vi "Main.vi"(11 "Module Admin":refnum<class "Delacor_lib_QMH_Module Admin.lvclass">) -> ()   [LabVIEW 2020, in "UI.lvlib"]
doc: "This template is based off of the Queued Message Handler design pattern and the Queued Message Handler project template that ships with LabVIEW.\n\nThe main difference is that the queue is private to this module and communication between modules is performed via Broadcast and Request events.\n\nRequest events are wrapped in public API methods and are handled in the Event Handling Loop (EHL) of this VI. Any module can register for Broadcast events sent by this module. The EHL generates messages based on user interface actions.\n\nThe Message Handling Loop (MHL) processes messages generated by the EHL, or by other messages. The messages are string values, so new messages can be added easily to the Message Cases case structure in the MHL. Each message cluster can also provide an optional value for Message Data, which is a variant that can be converted to whatever message-specific data is required.\n_____\nBased on Delacor QMH Project Template 5.0.0.82."
uses:
  UI.lvlib
  <vilib>/Delacor/Delacor QMH/Libraries/Module Admin_class/Delacor_lib_QMH_Module Admin.lvclass
  Module Data--cluster.ctl
  Stop Argument--cluster.ctl
  <vilib>/Delacor/Delacor QMH/Libraries/Message Queue_class/Delacor_lib_QMH_Message Queue.lvclass/Delacor_lib_QMH_Message Queue.ctl
  <vilib>/Delacor/Delacor QMH/Libraries/Module Admin_class/Delacor_lib_QMH_Module Admin.lvclass/Delacor_lib_QMH_Module Admin.ctl
  <vilib>/Utility/miscctls.llb/LVPointTypeDef.ctl
  <vilib>/Delacor/Delacor QMH/Libraries/Message Queue_class/Delacor_lib_QMH_Enqueue Message (Single).vi
  <vilib>/Delacor/Delacor QMH/Libraries/Module Admin_class/Delacor_lib_QMH_Get External Launch.vi
  <vilib>/Utility/error.llb/Error Cluster From Error Code.vi
  <vilib>/ErrorRing/Error Ring.xnode
  <vilib>/Delacor/Delacor QMH/Libraries/Message Queue_class/Delacor_lib_QMH_Message Queue.lvclass
  Acquisition whit helper loop/Acquisition whit helper loop.lvlib
panel:
  in  "Stop Acq":bool
  in  "Start Acq":bool
  out "error out":errorcluster
  out "Status":string
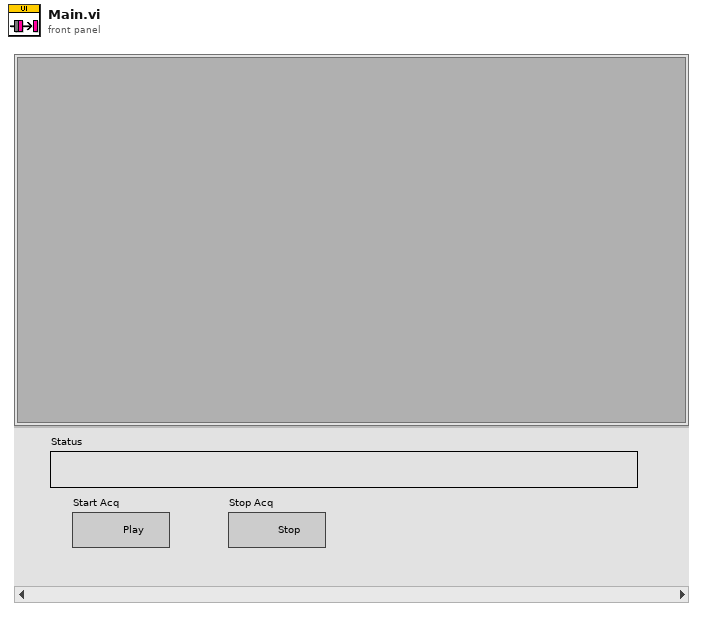
[diagram p1: front panel]
types:
  T1 = typedef "UI.lvlib/Request Events--cluster.ctl" = cluster{"Stop Module":refnum<user-event>, "Show Panel":refnum<user-event>, "Hide Panel":refnum<user-event>, "Get Module Execution Status":refnum<user-event>, "Show Diagram":refnum<user-event>}
  T2 = typedef "Acquisition whit helper loop.lvlib/Broadcast Events--cluster.ctl" = cluster{"Module Did Init":refnum<user-event>, "Status Updated":refnum<user-event>, "Error Reported":refnum<user-event>, "Module Did Stop":refnum<user-event>, "Update Module Execution Status":refnum<user-event>}
  T3 = typedef "UI.lvlib/Module Data--cluster.ctl" = cluster{"Status":string}
  T4 = enum32{"invalid lock state", "Not Locked", "Locked (No Password)", "Password-protected"}
  T5 = typedef "UI.lvlib/Stop Argument--cluster.ctl" = cluster{"Origin":string, "Exit via Stop Module Req?":bool, "Wait for Module to stop?":bool}
  T6 = enum32{"Invalid", "Standard", "Closed", "Hidden", "Minimized", "Maximized"}
  T7 = typedef "LVPointTypeDef.ctl" = cluster{"Horizontal":i16, "Vertical":i16}
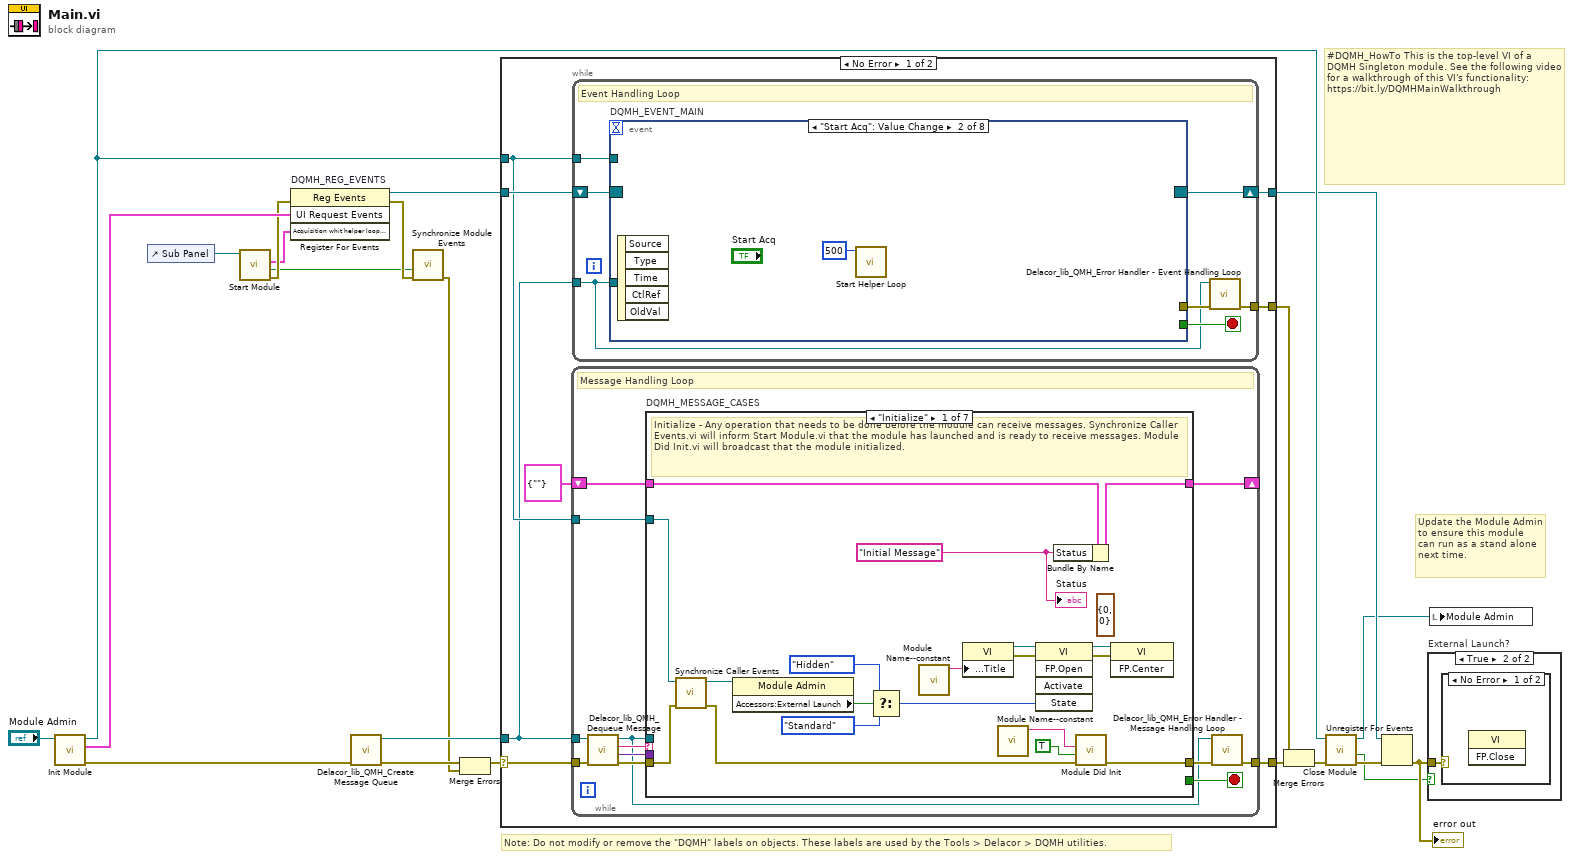
[diagram p0: block diagram]
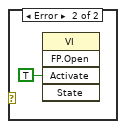
[diagram p3: hidden frame]
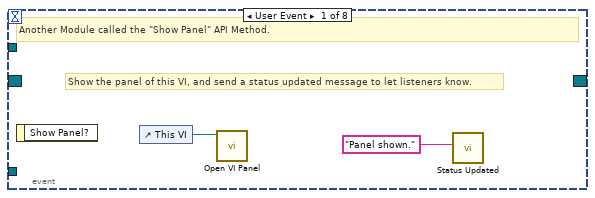
[diagram p4: hidden frame]
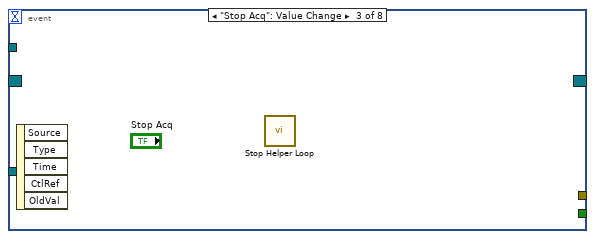
[diagram p5: hidden frame]
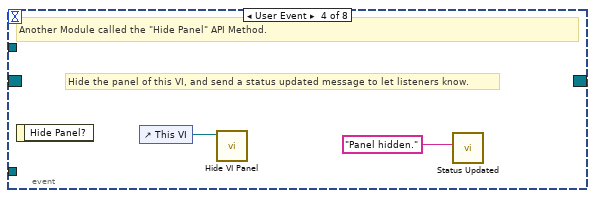
[diagram p6: hidden frame]
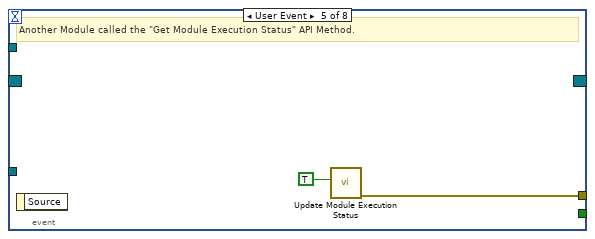
[diagram p7: hidden frame]
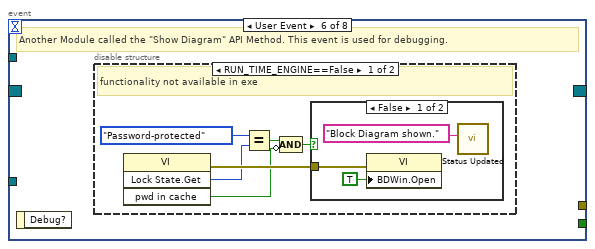
[diagram p8: hidden frame]
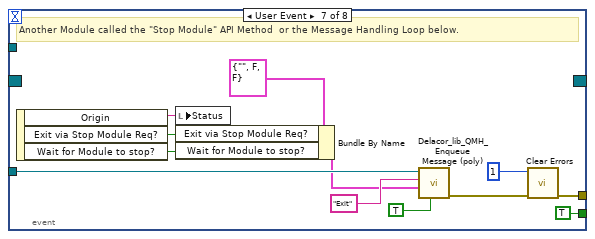
[diagram p11: hidden frame]
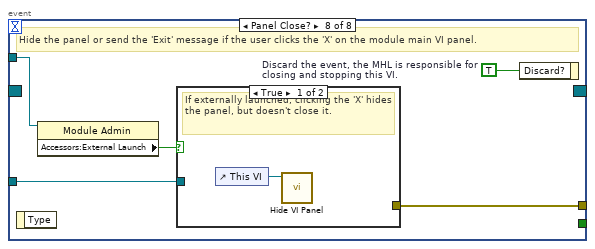
[diagram p12: hidden frame]
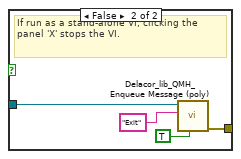
[diagram p13: hidden frame]
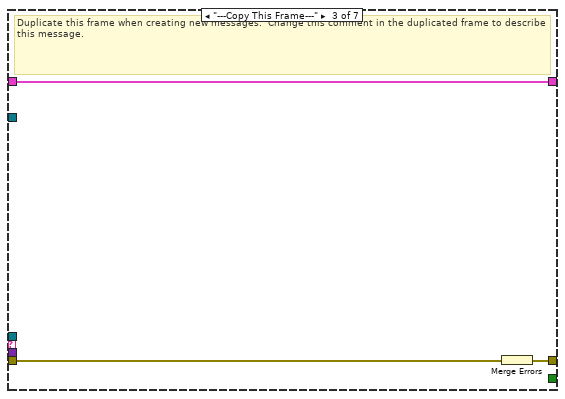
[diagram p15: hidden frame]
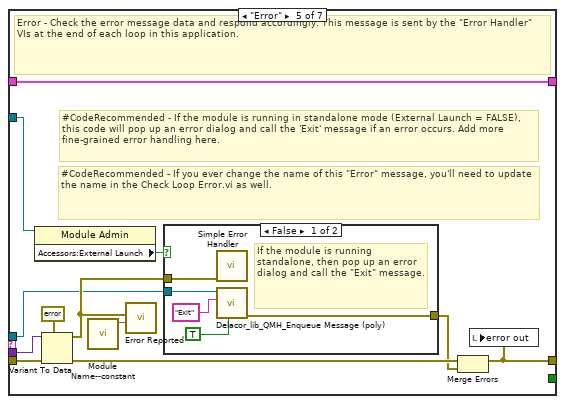
[diagram p17: hidden frame]
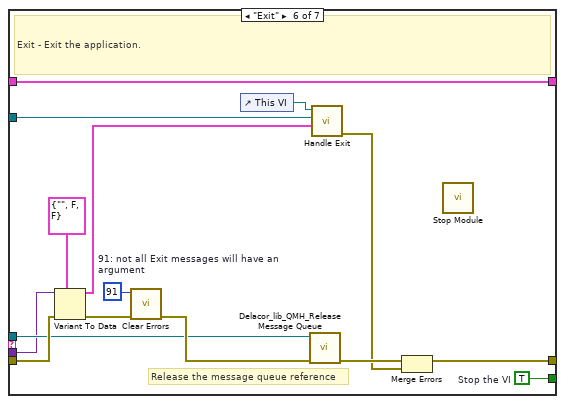
[diagram p19: hidden frame]
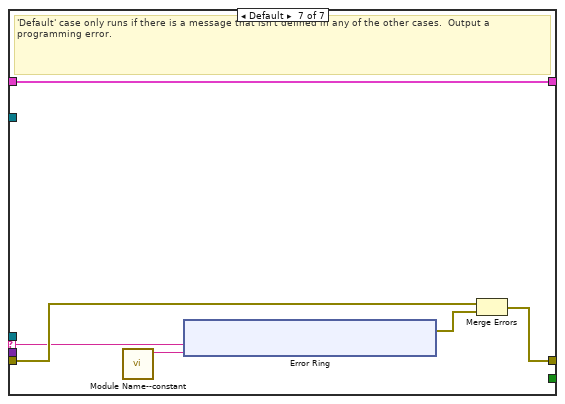
[diagram p20: hidden frame]
diagram:
  # "#DQMH_HowTo This is the top-level VI of a DQMH Singleton module. See the following video for a walkthrough of this VI's functionality: https://bit.ly/DQMHMainWalkthrough"
  # "Note: Do not modify or remove the \"DQMH\" labels on objects. These labels are used by the Tools > Delacor > DQMH utilities."
  # "Update the Module Admin to ensure this module can run as a stand alone next time."
  n1 = call "Init Module.vi"("Singleton Module Admin in"="Module Admin") -> ("error out"=w21:errorcluster, "UI Request Events"=w11:T1, "Singleton Module Admin out"=w14:refnum<class "Delacor_lib_QMH_Module Admin.lvclass">)  [unwired: 8 in]
  n2 = control-ref of="Sub Panel"() -> (w1:refnum<vi>)
  n3 = call "Start Module.vi"("Acquisition Panel"=w1) -> ("error out"=w4:errorcluster, "Wait for Event Sync?"=w3:bool, "Acquisition whit helper loop Broadcast Events"=w2:T2)  [unwired: 7 in, 1 out]
  n4 = register-events "DQMH_REG_EVENTS"(error in=w4, w11, w2) -> (reference out=w12:refnum<event-registration>, error out=w6:errorcluster)  [unwired: 1 in]
  n5 = call <vilib>:"Delacor_lib_QMH_Create Message Queue.vi"("error in (no error)"=w21) -> ("error out"=w16:errorcluster, "Message Queue"=w10:refnum<class "Delacor_lib_QMH_Message Queue.lvclass">)  [unwired: 9 in]
  n6 = call "Synchronize Module Events.vi"("error in (no error)"=w6, "Wait for Event Sync?"=w3) -> ("error out"=w5:errorcluster)  [unwired: 9 in]
  n7 = Merge Errors(w16, w5) -> (w15:errorcluster)
  n8 = case shown="No Error" w15 {
    selector: w15 -> [w28 w162]
    tunnel: [w30 w161] -> w22
    tunnel: [w27 w167] -> w13
    tunnel: w12 -> [w25 w167]
    tunnel: w10 -> [w23 w160]
    tunnel: [w29 _] -> w19
    tunnel: w14 -> [w24 w163]
    frame No Error {
      n9 = while {
        tunnel: w23 -> [w78]
        shift-right: [w82] -> _
        shift-left: T3 {"Status"=""} ("Data Cluster") -> [w83]
        tunnel: w28 -> [w86]
        tunnel: [w84] -> w30
        tunnel: w24 -> [w76]
        stop <- w81 stop-if-true
        # "Message Handling Loop"
        n10 = call-dynamic "Delacor_lib_QMH_Dequeue Message.vi"("error in (no error)"=w86, "Message Queue in"=w78) -> ("error out"=w85:errorcluster, "Message Data"=w79:variant, "Message"=w80:string, "Message Queue out"=w77:refnum<class "Delacor_lib_QMH_Message Queue.lvclass">)  [unwired: 6 in]
        n11 = case "DQMH_MESSAGE_CASES" shown="\"Initialize\"" w80 {
          selector: w80 -> [_ _ _ _ _ _ w147]
          tunnel: w77 -> [_ _ _ _ w117 w139 _]
          tunnel: w85 -> [w104 w108 w111 w113 w124 w145 w149]
          tunnel: [w102 w108 w110 w113 w120 w142 w150] -> w87
          tunnel: w83 -> [w94 w107 w109 w112 w119 w138 w148]
          tunnel: [w93 w107 w109 w112 w119 w138 w148] -> w82
          tunnel: [_ _ _ _ _ w137 _] -> w81
          tunnel: w79 -> [_ _ _ _ w118 w136 _]
          tunnel: w76 -> [w89 _ _ _ w116 w131 _]
          frame "Initialize" {
            (unwired) T7 {"Horizontal"=0, "Vertical"=0} ("Origin")
            w90 = "Initial Message" ("Initial Message")
            # "Initialize - Any operation that needs to be done before the module can receive messages. Synchronize Caller Events.vi will inform Start Module.vi that the module has launched and is ready to receive messages. Module Did Init.vi will broadcast that the module initialized."
            n12 = call "Synchronize Caller Events.vi"("error in (no error)"=w104, "Singleton Module Admin in"=w89) -> ("error out"=w103:errorcluster, "Singleton Module Admin out"=w88:refnum<class "Delacor_lib_QMH_Module Admin.lvclass">)  [unwired: 8 in]
            n13 = property class="Module Admin"(reference=w88) -> ("Accessors:External Launch"=w98:bool)  [unwired: 1 in, 2 out]
            n14 = Select(t=T6."Hidden" ("State"), s=w98, f=T6."Standard" ("State")) -> (s? t:f=w95:T6)
            n15 = call "Module Name--constant.vi"() -> ("Module Name"=w101:string)  [unwired: 11 in]
            n16 = property class="VI"("Front Panel.Title"=w101) -> (reference out=w100:refnum<vi>, error out=w106:errorcluster)  [unwired: 2 in]
            n17 = call "Module Name--constant.vi"() -> ("Module Name"=w91:string)  [unwired: 11 in]
            n18 = invoke class="VI" method="FP.Open"(reference=w100, error in=w106, "State"=w95) -> (reference out=w99:refnum<vi>, error out=w105:errorcluster)  [unwired: 2 in, 3 out]
            n19 = Bundle By Name(cluster=w94, "Status"=w90) -> (w93:T3)
            n20 = call "Module Did Init.vi"("error in (no error)"=w103, "Initialized?"=TRUE, "Origin"=w91) -> ("error out"=w102:errorcluster)  [unwired: 8 in]
            n21 = invoke class="VI" method="FP.Center"(reference=w99, error in=w105) -> ()  [unwired: 1 in, 3 out]
            "Status" <- w90
          }
          frame "--- Module Specific ---" {
            # "Separator -- The following cases handle messages specific to this Module."
          }
          frame "---Copy This Frame---" {
            # "Duplicate this frame when creating new messages.  Change this comment in the duplicated frame to describe this message."
            n22 = Merge Errors(w111) -> (w110:errorcluster)
          }
          frame "--- Exit and Error Handling---" {
            # "Separator - The following cases handle errors and exit messages."
          }
          frame "Error" {
            # "#CodeRecommended - If you ever change the name of this \"Error\" message, you'll need to update the name in the Check Loop Error.vi as well."
            # "#CodeRecommended - If the module is running in standalone mode (External Launch = FALSE), this code will pop up an error dialog and call the 'Exit' message if an error occurs. Add more fine-grained error handling here."
            # "Error - Check the error message data and respond accordingly. This message is sent by the \"Error Handler\" VIs at the end of each loop in this application."
            n23 = property class="Module Admin"(reference=w116) -> ("Accessors:External Launch"=w115:bool)  [unwired: 1 in, 2 out]
            n24 = Variant To Data(error in=w124, type=errorcluster {"status"=FALSE, "code"=0, "source"=""} ("error constant"), Variant=w118) -> (data=w125:errorcluster, error out=w122:errorcluster)
            n25 = call "Module Name--constant.vi"() -> ("Module Name"=w114:string)  [unwired: 11 in]
            n26 = call "Error Reported.vi"("Additional Information"=w114, "Error"=w125) -> ()  [unwired: 9 in, 1 out]
            n27 = case shown="False" w115 {
              tunnel: [w130 _] -> w121
              tunnel: w117 -> [w128 _]
              tunnel: w125 -> [w129 _]
              frame False {
                # "If the module is running standalone, then pop up an error dialog and call the \"Exit\" message."
                n28 = call <vilib>:"Simple Error Handler.vi"("error in (no error)"=w129) -> ()  [unwired: 4 in, 5 out]
                n29 = call-poly <vilib>:"Delacor_lib_QMH_Enqueue Message (poly).vi"("Priority Message? (F)"=TRUE, "Message"="Exit", "Message Queue in"=w128) -> ("error out"=w130:errorcluster)  [unwired: 7 in, 1 out]
              }
              frame True {
                # "If the module was launched externally, calling the Error Reported broadcast VI is the only action performed by the \"Error\" message. The module's caller can then process the error appropriately."
              }
            }
            n30 = Merge Errors(w122, w121) -> (w120:errorcluster)
            n31 = local write "error out"(w120) -> ()
          }
          frame "Exit" {
            w135 = 91  # 91: not all Exit messages will have an argument
            w137 = TRUE  # Stop the VI
            # "Release the message queue reference"
            # "Exit - Exit the application."
            n32 = Variant To Data(error in=w145, type=T5 {"Origin"="", "Exit via Stop Module Req?"=FALSE, "Wait for Module to stop?"=FALSE} ("Stop Argument"), Variant=w136) -> (data=w133:T5, error out=w141:errorcluster)
            n33 = call <vilib>:"Clear Errors.vi"("error in (no error)"=w141, "specific error code to clear (0: all)"=w135) -> ("error out"=w144:errorcluster)  [unwired: 4 in, 1 out]
            n34 = control-ref of="This VI"() -> (w132:refnum<vi>)
            n35 = call-dynamic "Delacor_lib_QMH_Release Message Queue.vi"("error in (no error)"=w144, "Message Queue"=w139) -> ("error out"=w143:errorcluster)  [unwired: 9 in]
            n36 = call "Handle Exit.vi"("Stop Argument"=w133, "Admin in"=w131, "VI reference"=w132) -> ("error out"=w140:errorcluster)  [unwired: 7 in, 1 out]
            n37 = Merge Errors(w143, w140) -> (w142:errorcluster)
            n38 = call "Stop Module.vi"() -> ()  [unwired: 11 in, 1 out]
          }
          frame Default {
            # "'Default' case only runs if there is a message that isn't defined in any of the other cases.  Output a programming error."
            n39 = call "Module Name--constant.vi"() -> ("Module Name"=w146:string)  [unwired: 11 in]
            n40 = xnode "Error Ring"("parameter 0"=w147, "parameter 1"=w146) -> ("error out"=w151:errorcluster)
            n41 = Merge Errors(w149, w151) -> (w150:errorcluster)
          }
        }
        n42 = call-dynamic "Delacor_lib_QMH_Error Handler - Message Handling Loop.vi"("error in (no error)"=w87, "Message Queue in"=w77) -> ("dup error in"=w84:errorcluster)  [unwired: 8 in, 1 out]
      }
      n43 = while {
        tunnel: w23 -> [w31]
        shift-right: [w34] -> w27
        shift-left: w25 -> [w35]
        tunnel: [w36] -> w29
        tunnel: w24 -> [w32]
        stop <- w33 stop-if-true
        # "Event Handling Loop"
        n44 = event "DQMH_EVENT_MAIN" shown="[1] \"Start Acq\": Value Change" {
          selector: w35 -> [_ _ _ _ _ _ _ _]
          dyn-events: [_ _ _ _ _ _ _ _] -> w34
          timeout: _ -> [_ _ _ _ _ _ _ _]
          tunnel: [_ _ _ _ _ _ TRUE ("Discard?") _] -> w33
          tunnel: w31 -> [_ _ _ _ _ _ w61 w68]
          tunnel: [_ _ _ _ w44 _ w64 w70] -> w37
          tunnel: w32 -> [_ _ _ _ _ _ _ w67]
          event User Event {
            # "Show the panel of this VI, and send a status updated message to let listeners know."
            # "Another Module called the \"Show Panel\" API Method."
            n45 = event-data() -> ()  [unwired: 1 in, 1 out]
            n46 = control-ref of="This VI"() -> (w39:refnum<vi>)
            n47 = call "Open VI Panel.vi"("VI"=w39) -> ()  [unwired: 10 in, 1 out]
            n48 = call "Status Updated.vi"("Status"="Panel shown." ("format string")) -> ()  [unwired: 10 in, 1 out]
          }
          event "Start Acq": Value Change {
            n49 = event-data() -> ()  [unwired: 1 in, 5 out]
            n50 = call "Start Helper Loop.vi"("Delay Timeout"=500) -> ()  [unwired: 10 in, 1 out]
          }
          event "Stop Acq": Value Change {
            n51 = event-data() -> ()  [unwired: 1 in, 5 out]
            n52 = call "Stop Helper Loop.vi"() -> ()  [unwired: 11 in, 1 out]
          }
          event User Event {
            # "Hide the panel of this VI, and send a status updated message to let listeners know."
            # "Another Module called the \"Hide Panel\" API Method."
            n53 = event-data() -> ()  [unwired: 1 in, 1 out]
            n54 = control-ref of="This VI"() -> (w42:refnum<vi>)
            n55 = call "Hide VI Panel.vi"("VI"=w42) -> ()  [unwired: 10 in, 1 out]
            n56 = call "Status Updated.vi"("Status"="Panel hidden." ("format string")) -> ()  [unwired: 10 in, 1 out]
          }
          event User Event {
            # "Another Module called the \"Get Module Execution Status\" API Method."
            n57 = event-data() -> ()  [unwired: 1 in, 1 out]
            n58 = call "Update Module Execution Status.vi"("Running?"=TRUE) -> ("error out"=w44:errorcluster)  [unwired: 10 in]
          }
          event User Event {
            # "Another Module called the \"Show Diagram\" API Method. This event is used for debugging."
            n59 = event-data() -> ()  [unwired: 1 in, 1 out]
            n60 = disable-structure shown="RUN_TIME_ENGINE==False" {
              frame condition #0 (active) {
                # "functionality not available in exe"
                n61 = invoke class="VI" method="Lock State.Get"() -> (error out=w50:errorcluster, "Get Lock State"=w49:T4, "pwd in cache"=w46:bool)  [unwired: 4 in, 1 out]
                n62 = Equal?(x=T4."Password-protected", y=w49) -> (x = y?=w47:bool)
                n63 = Compound Arithmetic op=AND(w47, invert w46) -> (w45:bool)
                n64 = case shown="False" w45 {
                  tunnel: w50 -> [w53 _]
                  frame False {
                    n65 = property class="VI"(error in=w53, "BDWin.Open"=TRUE ("Block Diagram Window:Open")) -> ()  [unwired: 1 in, 2 out]
                    n66 = call "Status Updated.vi"("Status"="Block Diagram shown." ("format string")) -> ()  [unwired: 10 in, 1 out]
                  }
                  frame True {
                    # "Password-protected VI, and the password is not in the cache. Do not show the diagram."
                  }
                }
              }
              frame condition #1 {
              }
            }
          }
          event User Event {
            # "Another Module called the \"Stop Module\" API Method  or the Message Handling Loop below."
            n67 = event-data() -> ("Origin"=w60:string, "Exit via Stop Module Req?"=w56:bool, "Wait for Module to stop?"=w55:bool)  [unwired: 1 in]
            n68 = local write "Status"(w60) -> ()
            n69 = Bundle By Name(cluster=T5 {"Origin"="", "Exit via Stop Module Req?"=FALSE, "Wait for Module to stop?"=FALSE} ("Stop Argument"), "Exit via Stop Module Req?"=w56, "Wait for Module to stop?"=w55) -> (w54:T5)
            n70 = call-poly <vilib>:"Delacor_lib_QMH_Enqueue Message (poly).vi"("Priority Message? (F)"=TRUE, "Message Data"=w54, "Message"="Exit", "Message Queue in"=w61) -> ("error out"=w65:errorcluster)  [unwired: 6 in, 1 out]
            n71 = call <vilib>:"Clear Errors.vi"("error in (no error)"=w65, "specific error code to clear (0: all)"=1) -> ("error out"=w64:errorcluster)  [unwired: 4 in, 1 out]
          }
          event Panel Close? {
            w69 = TRUE  # Discard the event, the MHL is responsible for closing and stopping this VI.
            # "Hide the panel or send the 'Exit' message if the user clicks the 'X' on the module main VI panel."
            n72 = event-data() -> ()  [unwired: 1 in, 1 out]
            n73 = property class="Module Admin"(reference=w67) -> ("Accessors:External Launch"=w66:bool)  [unwired: 1 in, 2 out]
            n74 = case shown="True" w66 {
              tunnel: w68 -> [_ w74]
              tunnel: [_ w75] -> w70
              frame True {
                # "If externally launched, clicking the 'X' hides the panel, but doesn't close it."
                n75 = control-ref of="This VI"() -> (w71:refnum<vi>)
                n76 = call "Hide VI Panel.vi"("VI"=w71) -> ()  [unwired: 10 in, 1 out]
              }
              frame False {
                # "If run as a stand-alone VI, clicking the panel 'X' stops the VI."
                n77 = call-poly <vilib>:"Delacor_lib_QMH_Enqueue Message (poly).vi"("Priority Message? (F)"=TRUE, "Message"="Exit", "Message Queue in"=w74) -> ("error out"=w75:errorcluster)  [unwired: 7 in, 1 out]
              }
            }
            n78 = event-data("Discard?"=w69) -> ()  [unwired: 1 in, 1 out]
          }
        }
        n79 = call-dynamic "Delacor_lib_QMH_Error Handler - Event Handling Loop.vi"("error in (no error)"=w37, "Message Queue in"=w31) -> ("dup error in"=w36:errorcluster)  [unwired: 8 in, 1 out]
      }
    }
    frame Error {
      # "Synchronize Caller Events.vi will inform Start Module.vi that the module has launched and will let the code calling Start Module.vi register for broadcasts and would permit the caller receive the broadcast that an error occurred at launch time."
      n80 = call-dynamic "Delacor_lib_QMH_Release Message Queue.vi"("error in (no error)"=w162, "Message Queue"=w160) -> ("error out"=w161:errorcluster)  [unwired: 9 in]
      n81 = call "Synchronize Caller Events.vi"("Singleton Module Admin in"=w163) -> ("error out"=w168:errorcluster)  [unwired: 9 in, 1 out]
      n82 = call "Module Name--constant.vi"() -> ("Module Name"=w166:string)  [unwired: 11 in]
      n83 = Format Into String(format string="An error occurred during initialization. %s is no longer running.", w166) -> (resulting string=w164:string)  [unwired: 2 in, 1 out]
      n84 = Merge Errors(w161, w168) -> (w169:errorcluster)
      n85 = call "Error Reported.vi"("Additional Information"=w164, "Error"=w169) -> ()  [unwired: 9 in, 1 out]
    }
  }
  n86 = Merge Errors(w19, w22) -> (w18:errorcluster)
  n87 = call "Close Module.vi"("error in (no error)"=w18, "Module Admin in"=w14) -> ("error out"=w20:errorcluster, "External Launch"=w7:bool, "Module Admin out"=w8:refnum<class "Delacor_lib_QMH_Module Admin.lvclass">)  [unwired: 7 in]
  n88 = Unregister For Events(event registration refnum=w13, error in=w20) -> (error out=w17:errorcluster)
  "error out" <- w17
  n89 = case "External Launch?" shown="True" w7 {
    tunnel: w17 -> [_ w170]
    frame False {
    }
    frame True {
      n90 = case shown="No Error" w170 {
        frame No Error {
          n91 = invoke class="VI" method="FP.Close"() -> ()  [unwired: 3 in, 3 out]
        }
        frame Error {
          n92 = invoke class="VI" method="FP.Open"("Activate"=TRUE ("Activate?")) -> ()  [unwired: 4 in, 5 out]
        }
      }
    }
  }
  n93 = local write "Module Admin"(w8) -> ()
